vi "Scanner-Barcode-Indentify_Test.vi"() -> ()   [LabVIEW 2019]
uses:
  <vilib>/myRIO/Instrument Drivers/Utilities/Utilities.lvlib
panel:
  out "辨識機率":dbl[](array[slide]) scale=0.0..10.0
  out "總辨識機率":i32[](graph)
  in  "Error In":errorcluster
  out "Error Out":errorcluster
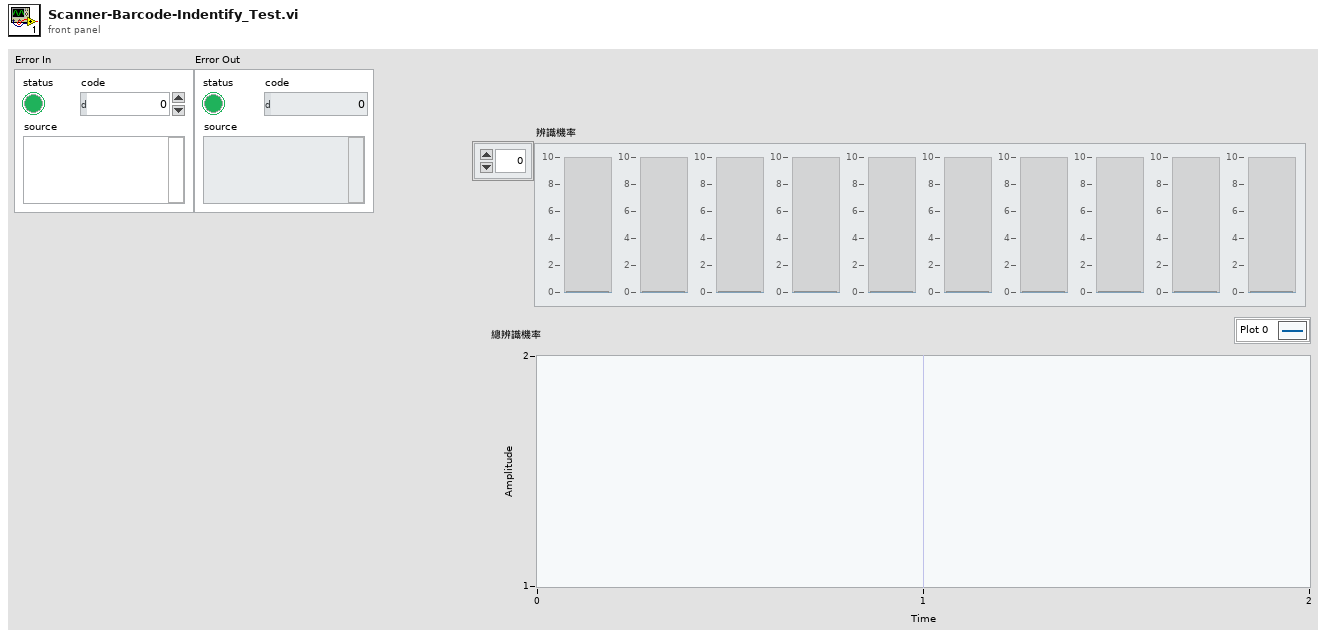
[diagram p1: front panel]
types:
  T1 = cluster{"對應顏色":enum16{"黃", "紅", "綠", "藍", "黑", "無"}, "對應顏色2":enum16{"黃", "紅", "綠", "藍", "黑", "無"}, "箱子位置":i32}[]
  T2 = cluster{"Array":i32[], "Array":i32[], "Array":i32[]}
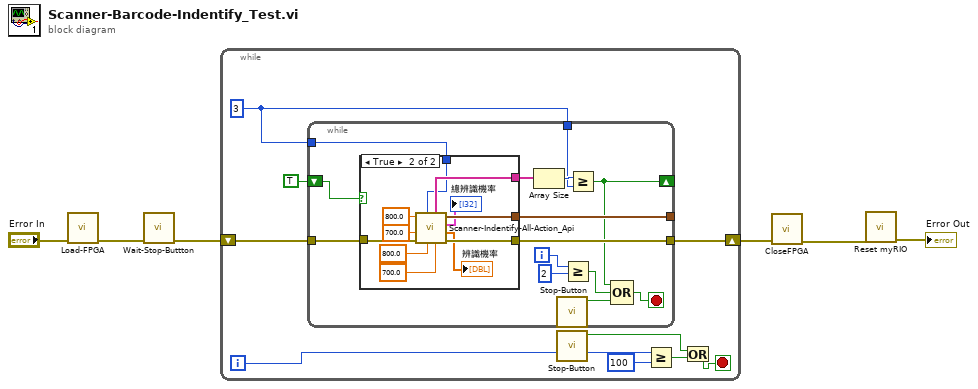
[diagram p0: block diagram]
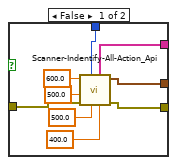
[diagram p2: hidden frame]
diagram:
  n1 = call "Load-FPGA.vi"("Error In"="Error In") -> ("Error Out"=w6:errorcluster)  [unwired: 10 in]
  n2 = call "Wait-Stop-Buttton.vi"("Error In"=w6) -> ("Error Out"=w2:errorcluster)  [unwired: 10 in]
  n3 = while {
    shift-right: [w14] -> w1
    shift-left: w2 -> [w15]
    i -> [w11]
    stop <- w9 stop-if-true
    w12 = 3 ("條碼數量")
    n4 = while {
      tunnel: w15 -> [w29]
      tunnel: [w26] -> w14
      tunnel: [w25] -> _
      shift-right: [w19] -> _
      shift-left: TRUE -> [w18]
      tunnel: w12 -> [w17]
      tunnel: w12 -> [w16]
      i -> [w24]
      stop <- w27 stop-if-true
      n5 = case shown="True" w18 {
        tunnel: w29 -> [w36 w49]
        tunnel: [w37 w48] -> w26
        tunnel: [w38 w47] -> w25
        tunnel: [w30 w46] -> w20
        tunnel: w17 -> [w31 w43]
        frame False {
          n6 = call "Scanner-Indentify-All-Action_Api.vi"("加速度 (回頭)"=400.0, "最高速 (回頭)"=500.0, "Barcode數量"=w31, "Error In"=w36, "加速度"=500.0, "最高速"=600.0) -> ("error out"=w37:errorcluster, "輸出顏色-位置"=w38:T1, "總辨識結果"=w30:string[])  [unwired: 1 in, 2 out]
        }
        frame True {
          n7 = call "Scanner-Indentify-All-Action_Api.vi"("加速度 (回頭)"=700.0, "最高速 (回頭)"=800.0, "Barcode數量"=w43, "Error In"=w49, "加速度"=700.0, "最高速"=800.0) -> ("error out"=w48:errorcluster, 1:"辨識機率"=→"辨識機率":dbl[], 2:"辨識機率"=→"總辨識機率":T2, "輸出顏色-位置"=w47:T1, "總辨識結果"=w46:string[])  [unwired: 1 in]
        }
      }
      n8 = Array Size(array=w20) -> (size(s)=w28:i32)
      n9 = call "Stop-Button.vi"() -> ("顯示按下?"=w21:bool)  [unwired: 10 in, 1 out]
      n10 = Greater Or Equal?(x=w24, y=2) -> (x >= y?=w22:bool)
      n11 = Greater Or Equal?(x=w28, y=w16) -> (x >= y?=w19:bool)
      n12 = Compound Arithmetic op=OR(w19, w22, w21) -> (w27:bool)
    }
    n13 = call "Stop-Button.vi"() -> ("顯示按下?"=w7:bool)  [unwired: 10 in, 1 out]
    n14 = Greater Or Equal?(x=w11, y=100) -> (x >= y?=w8:bool)
    n15 = Or(x=w7, y=w8) -> (x .or. y?=w9:bool)
  }
  n16 = call "CloseFPGA.vi"("Error In"=w1) -> ("Error Out"=w3:errorcluster)  [unwired: 10 in]
  n17 = call <vilib>:"Reset myRIO.vi"("error in (no error)"=w3) -> ("error out"=→"Error Out":errorcluster)  [unwired: 10 in]
